vi "Read All State Data.vi"(8 "error in (no error)":errorcluster, 11 "Framework Status in":refnum<class "Framework Status.lvclass">) -> (0 "error out":errorcluster, 2 "all state data":T1[](array[typedef]) {"period" format="%d us"; "duration" format="%d us"}, 3 "Framework Status out":refnum<class "Framework Status.lvclass">)   [LabVIEW 2019, in "DSF Core.lvlib" / "Framework Status.lvclass"]
uses:
  Framework Status.lvclass
  Status/Status Data.ctl
  Framework Status.lvclass/Framework Status.ctl
  Status/Status Pointer.lvclass
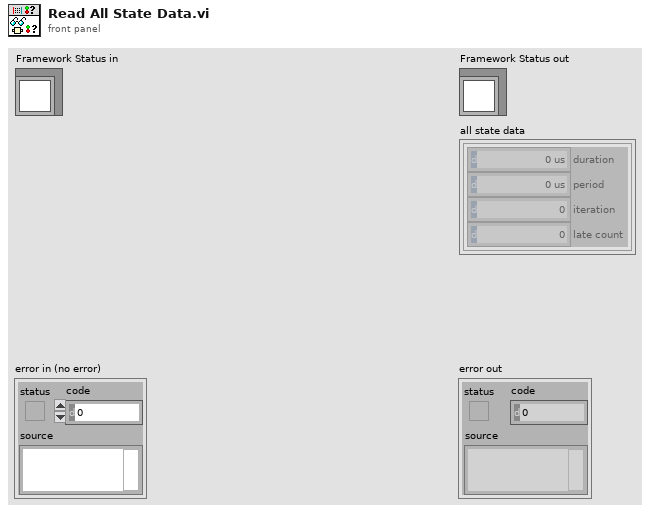
[diagram p1: front panel]
types:
  T1 = typedef "DSF Core.lvlib/Status Pointer.lvclass/Status Data.ctl" = cluster{"duration":u64, "period":u64, "iteration":u64, "late count":u64}
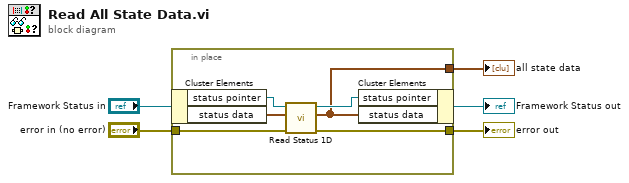
[diagram p0: block diagram]
diagram:
  n1 = in-place {
    in-place-border: "error in (no error)" -> [w8]
    in-place-border: [w6] -> w2
    in-place-border: [w7] -> w1
    n2 = in-place-cluster #1("Framework Status in") -> ("status pointer"=w11:refnum<class "Status Pointer.lvclass">, "status data"=w10:T1[])
    n3 = call "Read Status 1D.vi"("error in (no error)"=w8, "statuses in"=w10, "status pointer in"=w11) -> ("error out"=w6:errorcluster, "statuses out"=w7:T1[], "status pointer out"=w9:refnum<class "Status Pointer.lvclass">)  [unwired: 6 in]
    n4 = in-place-cluster #1("status pointer"=w9, "status data"=w7) -> (→"Framework Status out":refnum<class "Framework Status.lvclass">)
  }
  "error out" <- w2
  "all state data" <- w1
